vi "Calculate Ellipse Constants.vi"(0 "Center Coordinates":cluster{"x":dbl, "y":dbl}, 2 "Rotation Angle (rad)":dbl format="%#_13g", 3 "Semimajor Axis (a)":dbl format="%#_13g", 5 "Distance to Focus (c)":dbl format="%#_13g") -> (7 "Ellipse Constants":T1)   [LabVIEW 2013]
uses:
  <vilib>/Native 3D Graph/xcontrol/3DPC_SurfacePlot.xctl
  <vilib>/Analysis/baseanly.llb/A x Vector.vi
  <vilib>/gmath/NI_Gmath.lvlib
  <vilib>/Analysis/NI_AALBase.lvlib
panel:
  out "XY Graph":cluster{"X":dbl, "Y":dbl}[](graph)
  out "cos(x)":dbl
  out "Rotation Matrix":dbl[][](array[numeric])
  out "Semiminor Axis (b)":dbl
  out "b":dbl
  out "m":dbl
  out "y_min":dbl
  out "y_max":dbl
  out "xs":dbl[](array[numeric])
  out "f(x,y)":dbl[][](array[numeric])
  out "3D Graph":refnum<class "Base Datatype.lvclass">[](xcontrol)
  out "f":dbl
  in  "x_init":dbl
  out "Array":cluster{"x":dbl, "y":dbl}[](array[cluster])
  # "A x^2 + B xy + C y^2 + D x + E y + F = 0\nNote that this is the general equation of\nconic sections. An ellipse will have\nAC < 0 and cot 2*theta = (A-C)/B,\nwhere theta is the rotation angle."
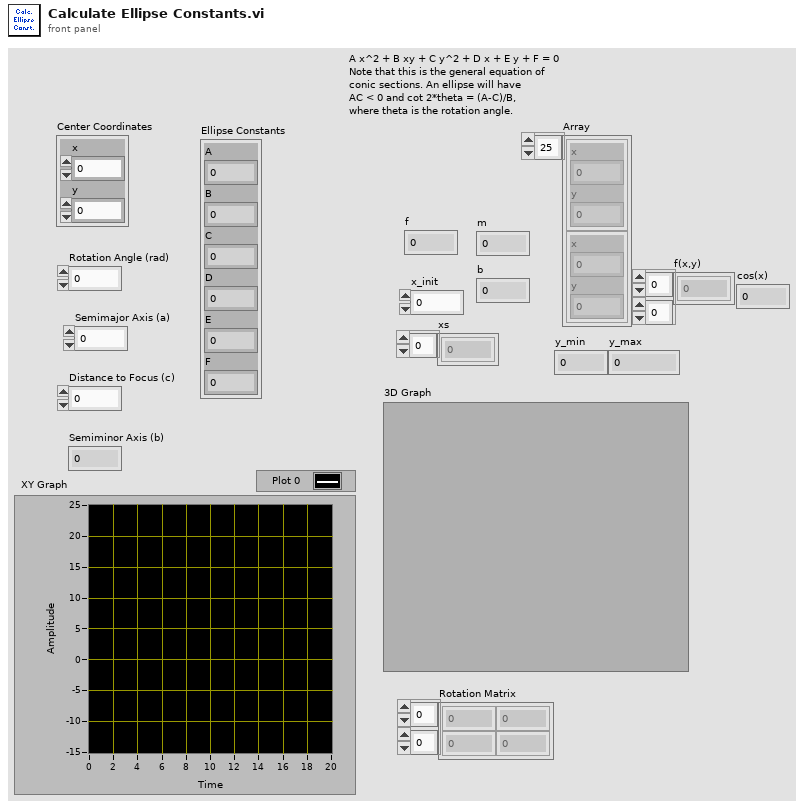
[diagram p1: front panel]
types:
  T1 = cluster{"A":dbl, "B":dbl, "C":dbl, "D":dbl, "E":dbl, "F":dbl}
  T2 = cluster{"A x Vector[0]":dbl, "A x Vector[1]":dbl}
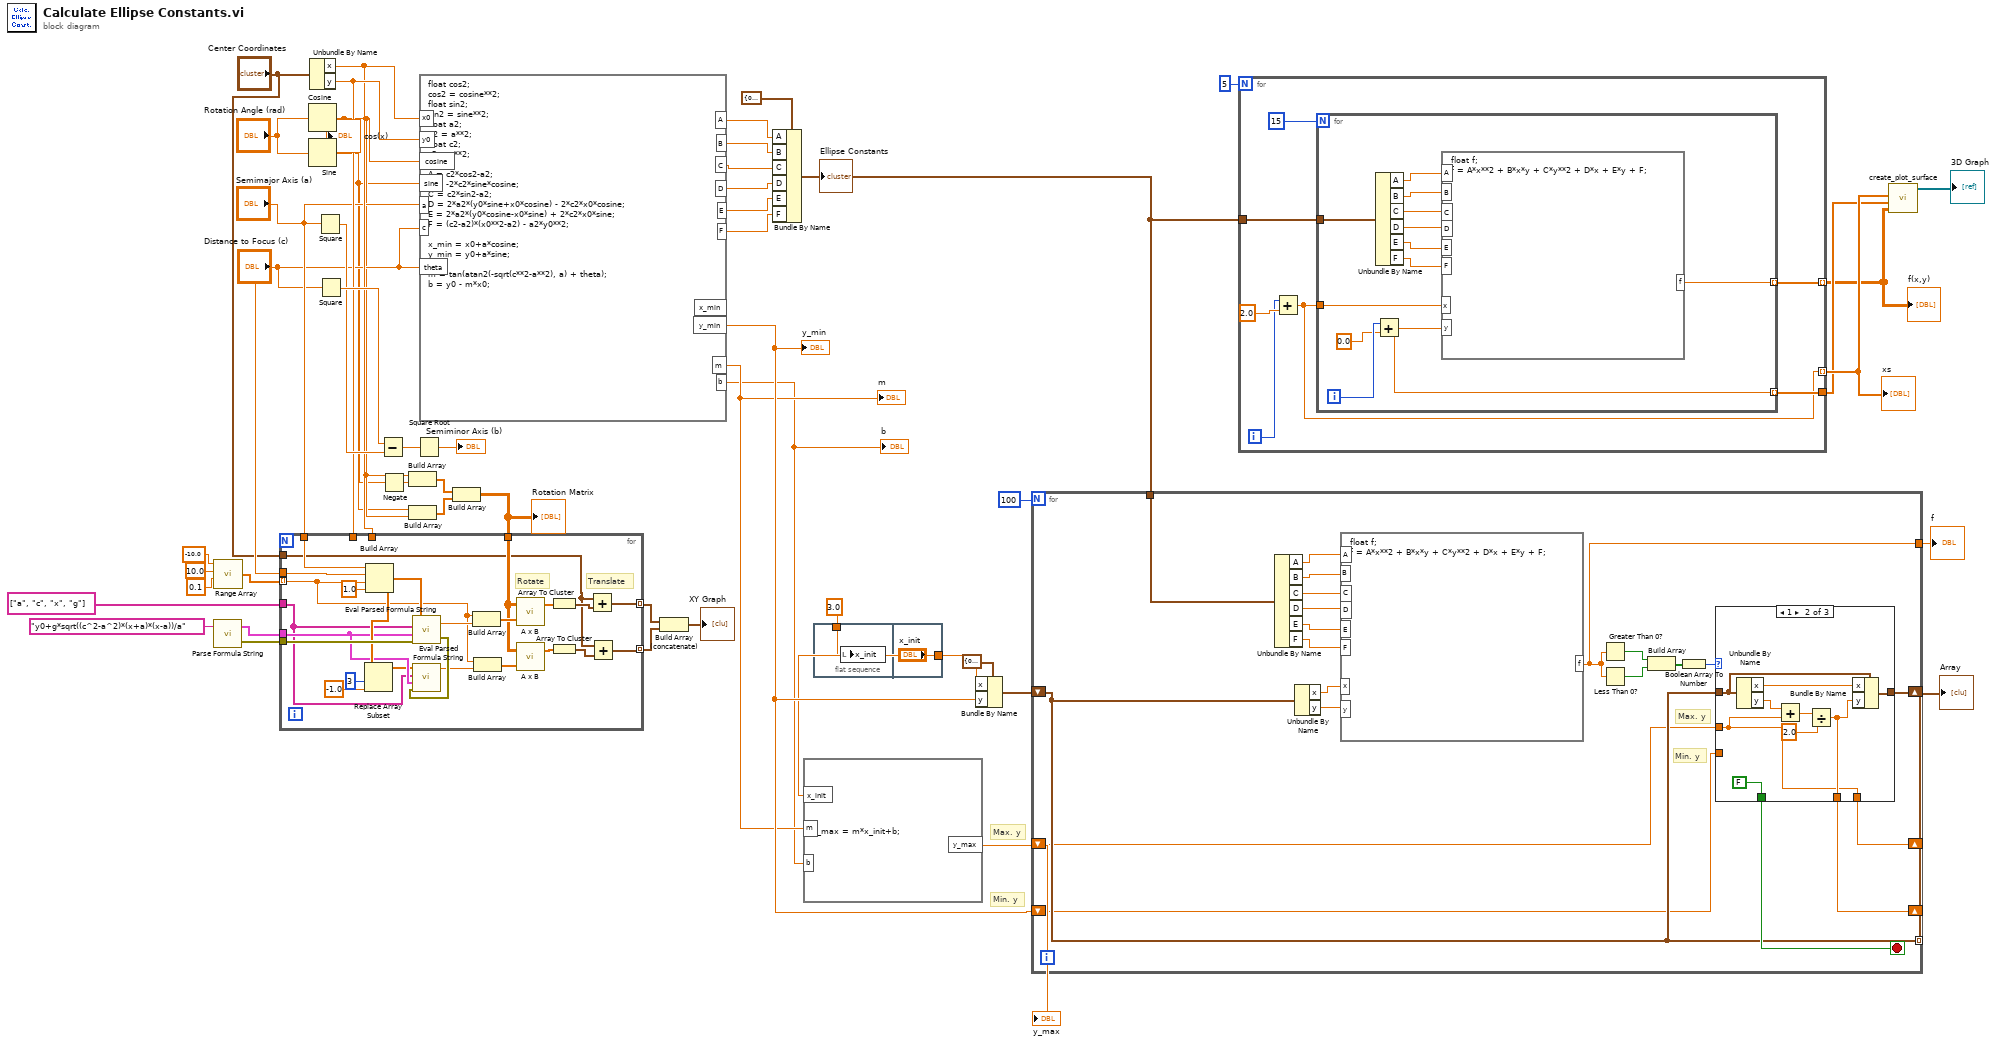
[diagram p0: block diagram]
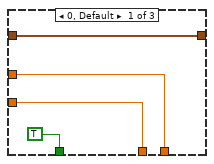
[diagram p2: hidden frame]
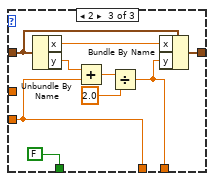
[diagram p3: hidden frame]
diagram:
  # "Max. y"
  # "Min. y"
  n1 = call <vilib>:"Parse Formula String.vi"("formula"="y0+g*sqrt((c^2-a^2)*(x+a)*(x-a))/a") -> ("error out"=w22:errorcluster, "Parsed Formula"=w20:cluster{"Table":i32[][], "Y Values":dbl[]})  [unwired: 1 in]
  n2 = call "Range Array.vi"("Step"=0.1, "Stop"=10.0, "Start"=-10.0) -> ("Range"=w16:dbl[])  [unwired: 3 in]
  n3 = Cosine(x="Rotation Angle (rad)") -> (cos(x)=w6:dbl)
  "cos(x)" <- w6
  n4 = Sine(x="Rotation Angle (rad)") -> (sin(x)=w5:dbl)
  n5 = Unbundle By Name("Center Coordinates") -> ("x"=w13:dbl, "y"=w14:dbl)
  n6 = Square(x="Semimajor Axis (a)") -> (x^2=w23:dbl)
  n7 = Square(x="Distance to Focus (c)") -> (x^2=w24:dbl)
  n8 = Subtract(x=w24, y=w23) -> (x-y=w26:dbl)
  n9 = Negate(x=w5) -> (-x=w10:dbl)
  n10 = Build Array(w6, w10) -> (w9:dbl[])
  n11 = Build Array(w5, w6) -> (w8:dbl[])
  n12 = Square Root(x=w26) -> (sqrt(x)=→"Semiminor Axis (b)":dbl)
  n13 = formula code="float cos2;\ncos2 = cosine**2;\nfloat sin2;\nsin2 = sine**2;\nfloat a2;\na2 = a**2;\nfloat c2;\nc2 = c**2;\n\nA = c2*cos2-a2;\nB = -2*c2*sine*cosine;\nC = c2*sin2-a2;\nD = 2*a2*(y0*sine+x0*cosine) - 2*c2*x0*cosine;\nE = 2*a2*(y0*cosine-x0*sine) + 2*c2*x0*sine;\nF = (c2-a2)*(x0**2-a2) - a2*y0**2;\n\nx_min = x0+a*cosine;\ny_min = y0+a*sine;\n\nm = tan(atan2(-sqrt(c**2-a**2), a) + theta);\nb = y0 - m*x0;"("x0"=w13, "y0"=w14, "cosine"=w6, "sine"=w5, "a"="Semimajor Axis (a)", "c"="Distance to Focus (c)", "theta"="Distance to Focus (c)") -> ("A"=w51:dbl, "B"=w50:dbl, "C"=w49:dbl, "D"=w48:dbl, "E"=w47:dbl, "F"=w46:dbl, "y_min"=w39:dbl, "m"=w38:dbl, "b"=w37:dbl)  [unwired: 1 out]
  "y_min" <- w39
  "m" <- w38
  "b" <- w37
  n14 = Build Array(w9, w8) -> (w7:dbl[][])
  "Rotation Matrix" <- w7
  n15 = for {
    tunnel: w22 -> [w75]
    tunnel: w20 -> [w67]
    tunnel: w16 -> [w59] mode=indexing
    tunnel: string[] ["a", "c", "x", "g"] ("Variables") -> [w66]
    tunnel: w14 -> [_]
    tunnel: w13 -> [_]
    tunnel: "Semimajor Axis (a)" -> [w74]
    tunnel: "Distance to Focus (c)" -> [w73]
    tunnel: w7 -> [w60]
    tunnel: [w52] -> w4 mode=indexing
    tunnel: [w53] -> w3 mode=indexing
    tunnel: "Center Coordinates" -> [w54]
    # "Translate"
    # "Rotate"
    n16 = Build Array(w74, w73, w59, 1.0 ("element")) -> (w71:dbl[])
    n17 = Replace Array Subset(array=w71, new element=-1.0 ("new element/subarray"), index=3) -> (w65:dbl[])
    n18 = call <vilib>:"Eval Parsed Formula String.vi"("error in (no error)"=w75, "Parsed Formula"=w67, "Variables"=w66, "X Values"=w71) -> ("error out"=w68:errorcluster, "y value"=w64:dbl)
    n19 = call <vilib>:"Eval Parsed Formula String.vi"("error in (no error)"=w68, "Parsed Formula"=w67, "Variables"=w66, "X Values"=w65) -> ("y value"=w63:dbl)  [unwired: 1 out]
    n20 = Build Array(w59, w64) -> (w62:dbl[])
    n21 = Build Array(w59, w63) -> (w61:dbl[])
    n22 = call-poly <vilib>:"A x B.vi"("Vector"=w62, "A"=w60) -> ("A x Vector"=w58:dbl[])  [unwired: 1 out]
    n23 = call-poly <vilib>:"A x B.vi"("Vector"=w61, "A"=w60) -> ("A x Vector"=w57:dbl[])  [unwired: 1 out]
    n24 = Array To Cluster(array=w58) -> (cluster=w56:T2)
    n25 = Array To Cluster(array=w57) -> (cluster=w55:T2)
    n26 = Add(x=w54, y=w56) -> (x+y=w52:cluster{dbl, dbl})
    n27 = Add(x=w54, y=w55) -> (x+y=w53:cluster{dbl, dbl})
  }
  n28 = Build Array (concatenate)(w4, w3) -> (→"XY Graph":cluster{dbl, dbl}[])
  n29 = Bundle By Name(cluster=T1 {"A"=0.0, "B"=0.0, "C"=0.0, "D"=0.0, "E"=0.0, "F"=0.0} ("Ellipse Constants"), "A"=w51, "B"=w50, "C"=w49, "D"=w48, "E"=w47, "F"=w46) -> (w32:T1)
  "Ellipse Constants" <- w32
  n30 = formula code="y_max = m*x_init+b;"("x_init"=w35, "m"=w38, "b"=w37) -> ("y_max"=w36:dbl)
  "y_max" <- w36
  n31 = flat-sequence {
    tunnel: 3.0 ("x_min") -> [w76]
    tunnel: ["x_init"] -> w35
    frame #0 {
      n32 = local write "x_init"(w76) -> ()
    }
    frame #1 {
    }
  }
  n33 = Bundle By Name(cluster=cluster{"x":dbl, "y":dbl} {"x"=0.0, "y"=0.0} ("Center Coordinates"), "x"=w35, "y"=w39) -> (w40:cluster{"x":dbl, "y":dbl})
  n34 = for {
    N: 100 -> [_]
    shift-right: [w85] -> _
    shift-left: w40 -> [w83]
    tunnel: w32 -> [w92]
    tunnel: [w83] -> w43 mode=indexing
    shift-right: [w80] -> _
    shift-left: w39 -> [w81]
    shift-right: [w79] -> _
    shift-left: w36 -> [w82]
    tunnel: [w78] -> w34
    stop <- w84 stop-if-true
    # "Min. y"
    # "Max. y"
    n35 = Unbundle By Name(w92) -> ("A"=w98:dbl, "B"=w97:dbl, "C"=w96:dbl, "D"=w95:dbl, "E"=w94:dbl, "F"=w93:dbl)
    n36 = Unbundle By Name(w83) -> ("x"=w91:dbl, "y"=w90:dbl)
    n37 = formula code="float f;\nf = A*x**2 + B*x*y + C*y**2 + D*x + E*y + F;"("A"=w98, "B"=w97, "C"=w96, "D"=w95, "E"=w94, "F"=w93, "x"=w91, "y"=w90) -> ("f"=w78:dbl)
    n38 = Greater Than 0?(x=w78) -> (x > 0?=w89:bool)
    n39 = Less Than 0?(x=w78) -> (x < 0?=w88:bool)
    n40 = Build Array(w89, w88) -> (w87:bool[])
    n41 = Boolean Array To Number(Boolean array=w87) -> (number=w86:u32)
    n42 = case shown="1" w86 {
      tunnel: w83 -> [w102 w106 w118]
      tunnel: [w102 w105 w119] -> w85
      tunnel: [TRUE FALSE FALSE] -> w84
      tunnel: w82 -> [w100 w103 _]
      tunnel: w81 -> [w99 _ w112]
      tunnel: [w99 w104 w112] -> w80
      tunnel: [w100 w103 w113] -> w79
      frame 0, Default {
      }
      frame 1 {
        n43 = Unbundle By Name(w106) -> ("x"=w110:dbl, "y"=w109:dbl)
        n44 = Add(x=w109, y=w103) -> (x+y=w108:dbl)
        n45 = Divide(x=w108, y=2.0) -> (x/y=w104:dbl)
        n46 = Bundle By Name(cluster=w106, "x"=w110, "y"=w104) -> (w105:cluster{"x":dbl, "y":dbl})
      }
      frame 2 {
        n47 = Unbundle By Name(w118) -> ("x"=w117:dbl, "y"=w116:dbl)
        n48 = Add(x=w116, y=w112) -> (x+y=w115:dbl)
        n49 = Divide(x=w115, y=2.0) -> (x/y=w113:dbl)
        n50 = Bundle By Name(cluster=w118, "x"=w117, "y"=w113) -> (w119:cluster{"x":dbl, "y":dbl})
      }
    }
  }
  "Array" <- w43
  "f" <- w34
  n51 = for {
    N: 5 -> [_]
    tunnel: w32 -> [w127]
    tunnel: [w121] -> w30 mode=indexing
    tunnel: [w125] -> w29
    tunnel: [w124] -> w28 mode=indexing
    i -> [w122]
    n52 = Add(x=w122, y=2.0) -> (x+y=w121:dbl)
    n53 = for {
      N: 15 -> [_]
      tunnel: w127 -> [w133]
      tunnel: [w131] -> w125 mode=indexing
      tunnel: [w130] -> w124 mode=indexing
      tunnel: w121 -> [w128]
      i -> [w132]
      n54 = Add(x=w132, y=0.0) -> (x+y=w131:dbl)
      n55 = Unbundle By Name(w133) -> ("A"=w139:dbl, "B"=w138:dbl, "C"=w137:dbl, "D"=w136:dbl, "E"=w135:dbl, "F"=w134:dbl)
      n56 = formula code="float f;\nf = A*x**2 + B*x*y + C*y**2 + D*x + E*y + F;"("A"=w139, "B"=w138, "C"=w137, "D"=w136, "E"=w135, "F"=w134, "x"=w128, "y"=w131) -> ("f"=w130:dbl)
    }
  }
  "f(x,y)" <- w28
  "xs" <- w30
  n57 = call <vilib>:"create_plot_surface.vi"("z matrix"=w28, "y vector"=w29, "x vector"=w30) -> ("plots out"=→"3D Graph":refnum<class "Base Datatype.lvclass">[])  [unwired: 2 in, 6 out]
